vi "video player.vi"() -> ()   [LabVIEW 2020]
panel:
  in  "Path":path
  in  "WindowsMediaPlayer":refnum<k7>(container)
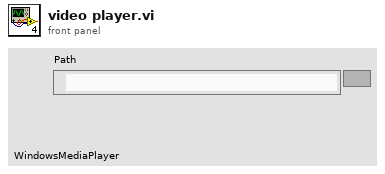
[diagram p1: front panel]
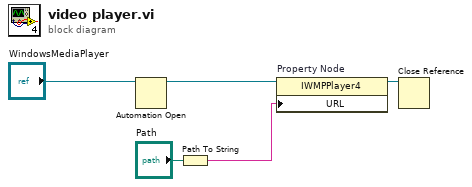
[diagram p0: block diagram]
diagram:
  n1 = Automation Open(Automation Refnum="WindowsMediaPlayer") -> (Automation Refnum=w4:refnum<k7>)  [unwired: 3 in, 1 out]
  n2 = Path To String(path="Path") -> (string=w1:string)
  n3 = property on="Property Node" class="IWMPPlayer4"(reference=w4, "URL"=w1) -> (reference out=w3:refnum<k7>)  [unwired: 1 in, 1 out]
  n4 = Close Reference(reference=w3) -> ()  [unwired: 1 in, 1 out]
